vi "Find and Rename Libraries.vi"(0 "Owned Items[]":refnum<vi>[](array[refnum]), 2 "Private Data.Application Ref":refnum<vi>, 5 "new name":string, 7 "name to replace":string, 11 "error in":errorcluster) -> (15 "error out":errorcluster)   [LabVIEW 2018, in "Springboard TLB`.lvlib"]
uses:
  Springboard TLB`.lvlib
  <vilib>/regexp/Match Regular Expression.xnode
panel:
  out "Array 2":string[](array[string])
  out "Array":string[](array[string])
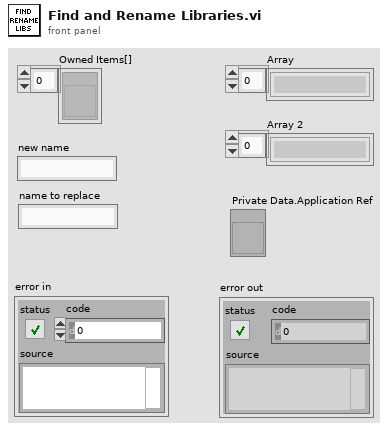
[diagram p1: front panel]
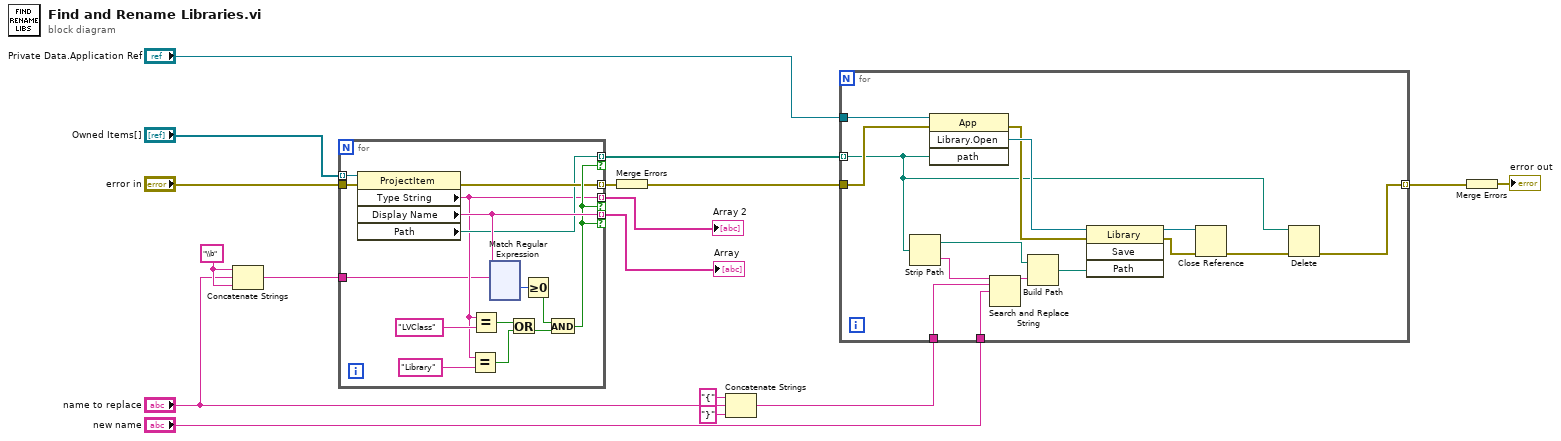
[diagram p0: block diagram]
diagram:
  w5 = "\\b" ("string")
  n1 = Concatenate Strings(w5, "name to replace", w5) -> (w6:string)
  n2 = for {
    tunnel: "Owned Items[]" -> [w32] mode=indexing
    tunnel: [w20] -> w12 mode=indexing if=w28
    tunnel: [w30] -> w13 mode=indexing if=w28
    tunnel: [w24] -> w7 mode=indexing if=w28
    tunnel: [w27] -> w16 mode=indexing
    tunnel: "error in" -> [w26]
    tunnel: w6 -> [w18]
    n3 = property class="ProjectItem"(reference=w32, error in=w26) -> (error out=w27:errorcluster, "Type String"=w20:string, "Display Name"=w30:string, "Path"=w24:path)  [unwired: 1 out]
    n4 = Equal?(x=w20, y="Library") -> (x = y?=w19:bool)
    n5 = Equal?(x=w20, y="LVClass") -> (x = y?=w22:bool)
    n6 = xnode "Match Regular Expression"("input string"=w30, "regular expression"=w18) -> ("offset past match"=w29:i32)  [unwired: 4 in, 4 out]
    n7 = Or(x=w22, y=w19) -> (x .or. y?=w23:bool)
    n8 = Greater Or Equal To 0?(x=w29) -> (x >= 0?=w25:bool)
    n9 = And(x=w25, y=w23) -> (x .and. y?=w28:bool)
  }
  "Array" <- w13
  "Array 2" <- w12
  n10 = Merge Errors(w16) -> (w17:errorcluster)
  n11 = Concatenate Strings("{" ("string"), "name to replace", "}" ("string")) -> (w1:string)
  n12 = for {
    tunnel: "Private Data.Application Ref" -> [w161]
    tunnel: w7 -> [w148] mode=indexing
    tunnel: w17 -> [w160]
    tunnel: [w149] -> w10 mode=indexing
    tunnel: "new name" -> [w151]
    tunnel: w1 -> [w147]
    n13 = Strip Path(path=w148) -> (stripped path=w152:path, name=w154:string)
    n14 = invoke class="App" method="Library.Open"(reference=w161, error in=w160, "path"=w148) -> (error out=w158:errorcluster, "Open Library"=w159:refnum<vi>)  [unwired: 1 in, 2 out]
    n15 = Search and Replace String(input string=w154, search string=w147, replace string=w151) -> (result string=w153:string)  [unwired: 5 in, 3 out]
    n16 = Build Path(base path=w152, name or relative path=w153) -> (appended path=w150:path)
    n17 = invoke class="Library" method="Save"(reference=w159, error in=w158, "Path"=w150) -> (reference out=w156:refnum<vi>, error out=w157:errorcluster)  [unwired: 1 in, 2 out]
    n18 = Close Reference(reference=w156, error in (no error)=w157) -> (error out=w155:errorcluster)
    n19 = Delete(path (use dialog)=w148, error in=w155) -> (error out=w149:errorcluster)  [unwired: 3 in, 2 out]
  }
  n20 = Merge Errors(w10) -> (→"error out":errorcluster)
